vi "pushBack.vi"(8 "error in (no error)":errorcluster, 10 "Object in":refnum<class "IBaseObject.lvclass">, 11 "IList in":refnum<class "IList.lvclass">) -> (0 "error out":errorcluster, 2 "Object out":refnum<class "IBaseObject.lvclass">, 3 "IList out":refnum<class "IList.lvclass">)   [LabVIEW 2022 SP3, in "openDAQ.lvlib" / "daqCoreTypes.lvlib" / "IList.lvclass"]
uses:
  <instrlib>/openDAQ/Public/Classes/daqCoreTypes/IList/IList.lvclass
  C:/Program Files (x86)/National Instruments/LabVIEW 2022/instr.lib/openDAQ/Public/Classes/IBaseObject/IBaseObject.lvclass
  <instrlib>/openDAQ/Public/Classes/IBaseObject/IBaseObject.lvclass/IBaseObject.ctl
  <instrlib>/openDAQ/Public/Classes/IBaseObject/Accessor/Read reference.vi
  <instrlib>/openDAQ/Public/Classes/IBaseObject/Accessor/Write reference.vi
  <instrlib>/openDAQ/Public/Classes/daqCoreTypes/IList/IList.lvclass/IList.ctl
  <instrlib>/openDAQ/Public/Classes/IBaseObject/IBaseObject.lvclass
  <instrlib>/openDAQ/Binaries/Windows/x86/copendaq32.dll
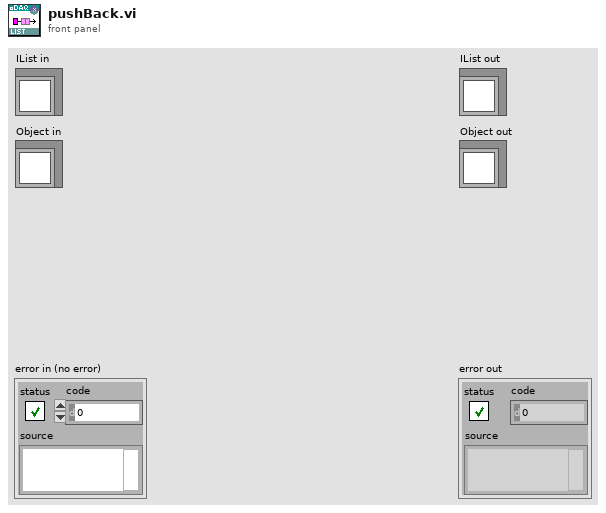
[diagram p1: front panel]
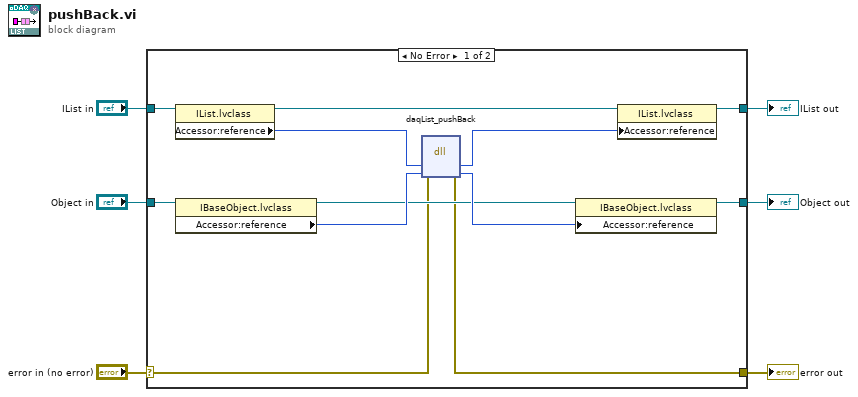
[diagram p0: block diagram]
diagram:
  n1 = case shown="No Error" "error in (no error)" {
    selector: "error in (no error)" -> [w8 w21]
    tunnel: [w7 w21] -> w5
    tunnel: [w16 w20] -> w3
    tunnel: "IList in" -> [w18 w20]
    tunnel: "Object in" -> [w13 w19]
    tunnel: [w9 w19] -> w1
    frame No Error {
      n2 = property class="IList.lvclass"(reference=w18) -> (reference out=w17:refnum<class "IList.lvclass">, "Accessor:reference"=w15:i64)  [unwired: 1 in, 1 out]
      n3 = property class="IBaseObject.lvclass"(reference=w13) -> (reference out=w10:refnum<class "IBaseObject.lvclass">, "Accessor:reference"=w12:i64)  [unwired: 1 in, 1 out]
      n4 = dll-call lib="C:/Program Files (x86)/National Instruments/LabVIEW 2022/instr.lib/openDAQ/Binaries/Windows/x86/copendaq*.*" fn="daqList_pushBack"(error in=w8, "daqList"=w15, "object"=w12) -> (error out=w7:errorcluster, "daqList"=w14:i64, "object"=w11:i64)  [unwired: 3 in, 1 out]
      n5 = property class="IBaseObject.lvclass"(reference=w10, "Accessor:reference"=w11) -> (reference out=w9:refnum<class "IBaseObject.lvclass">)  [unwired: 1 in, 1 out]
      n6 = property class="IList.lvclass"(reference=w17, "Accessor:reference"=w14) -> (reference out=w16:refnum<class "IList.lvclass">)  [unwired: 1 in, 1 out]
    }
    frame Error {
    }
  }
  "error out" <- w5
  "IList out" <- w3
  "Object out" <- w1
